vi "Get Coordinates.vi"(8 "error in (no error)":errorcluster, 9 "Plot ID":i32, 11 "3D Waterfall.lvclass in":refnum<class "3D Waterfall.lvclass">) -> (0 "error out":errorcluster, 1 "Coordinates System":enum16{"Cartesian", "Cylindrical", "Spherical"}(ring), 3 "3D Waterfall.lvclass out":refnum<class "3D Waterfall.lvclass">)   [LabVIEW 2017, in "3D Waterfall.lvclass"]
uses:
  <vilib>/Math Plots/3D Math Plots/3D Waterfall/3D Waterfall/3D Waterfall.lvclass
  <vilib>/Math Plots/3D Math Plots/3D Waterfall/3D Waterfall/3D Waterfall.lvclass/3D Waterfall.ctl
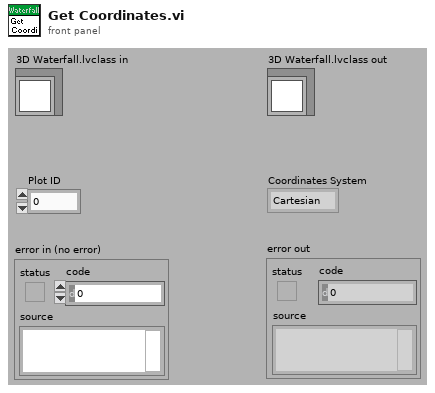
[diagram p1: front panel]
types:
  T1 = typedef "3D Waterfall.lvclass/3D Waterfall Propery Array.ctl" = T2[]
  T2 = typedef "3D Waterfall.lvclass/3D Waterfall Property.ctl" = cluster{"General Property":cluster{"Plot Name":string, "Coordinate System":enum16{"Cartesian", "Cylindrical", "Spherical"}, "Opacity":sgl}, "Projection Property":cluster{"Draw XY":bool, "Draw YZ":bool, "Draw XZ":bool}, "Plot Property":cluster{"Line Style":T3, "Line Width":sgl, "Color Ramp Cluster":T4, "Antialiasing":bool}, "Waterfall Property":cluster{"Waterfall Mode":enum16{"Lines", "Slices"}}}
  T3 = typedef "3D Plot.lvclass/Line Type.ctl" = enum16{"None", "Solid", "Dash", "Dot", "Dash Dot"}
  T4 = typedef "3D Plot.lvclass/Color Ramp Cluster.ctl" = cluster{"Color Ramp Style":enum16{"None", "Shaded", "Color spectrum", "Grey scale", "Custom"}, "Color Ramp Array":u32[], "Color Ramp Index":i32[], "Interpolate?":bool, "Logarithm?":bool}
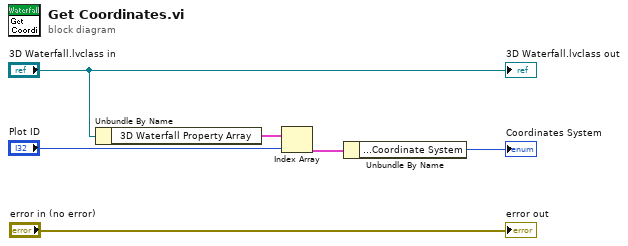
[diagram p0: block diagram]
diagram:
  n1 = Unbundle By Name("3D Waterfall.lvclass in") -> ("3D Waterfall Property Array"=w6:T1)
  n2 = Index Array(array=w6, index="Plot ID") -> (element=w5:T2)
  n3 = Unbundle By Name(w5) -> ("General Property.Coordinate System"=→"Coordinates System":enum16{"Cartesian", "Cylindrical", "Spherical"})
  "3D Waterfall.lvclass out" <- "3D Waterfall.lvclass in"
  "error out" <- "error in (no error)"
